vi "ServerGlobalVariables.vi"() -> ()   [LabVIEW 2025]
panel:
  in  "Teams":set{u32}[](array[numeric])
  in  "Empty Team Slots":set{u8}(c389)
  in  "PlayerInfoMap":T1(c390)
  in  "PlayerIDConnectionMap":map{u32, cluster{"Address":u32, "Port":u16}}(c390)
  in  "PlayerConnectionIDMap":map{cluster{"Address":u32, "Port":u16}, u32}(c390)
  out "ID Counter":u32
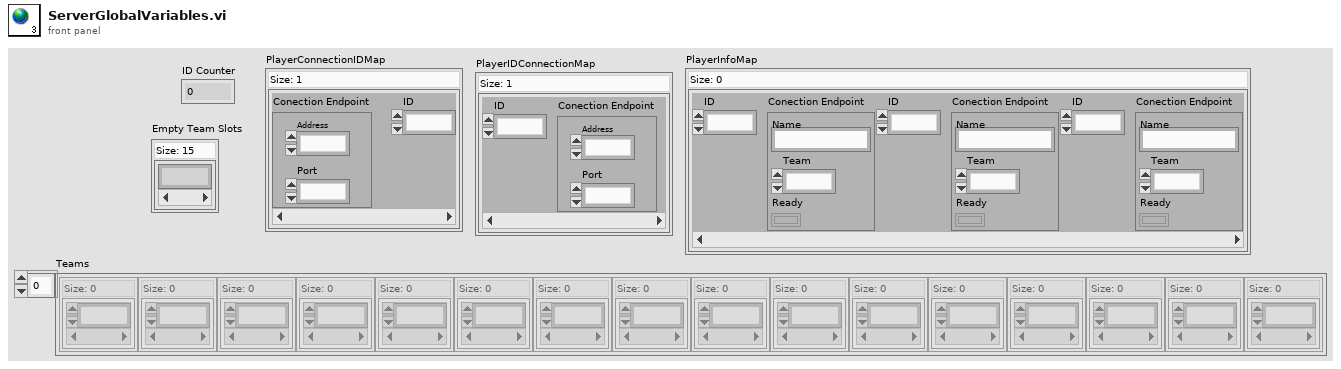
[diagram p1: front panel]
types:
  T1 = map{u32, cluster{"Name":string, "Team":u8, "Ready":bool}}
diagram:
